vi "分层图显示1.1.vi"(11 "IN":string) -> (3 "OUT":string)   [LabVIEW 2016]
uses:
  <vilib>/Utility/file.llb/Read Delimited Spreadsheet (DBL).vi
panel:
  out "导入进度":u8(slide) scale=0.0..100.0
  in  "min":dbl format="%#_4e"
  in  "max":dbl format="%#_4e"
  in  "ESC":bool
  out "分层图":dbl[][](graph)
  in  "NEXT":bool
  in  "层数:":i32
  out "数组":dbl[][][](array[numeric])
  # "强度表"
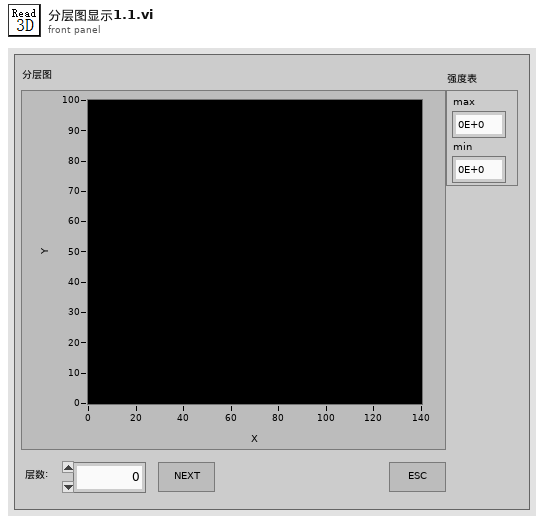
[diagram p1: front panel]
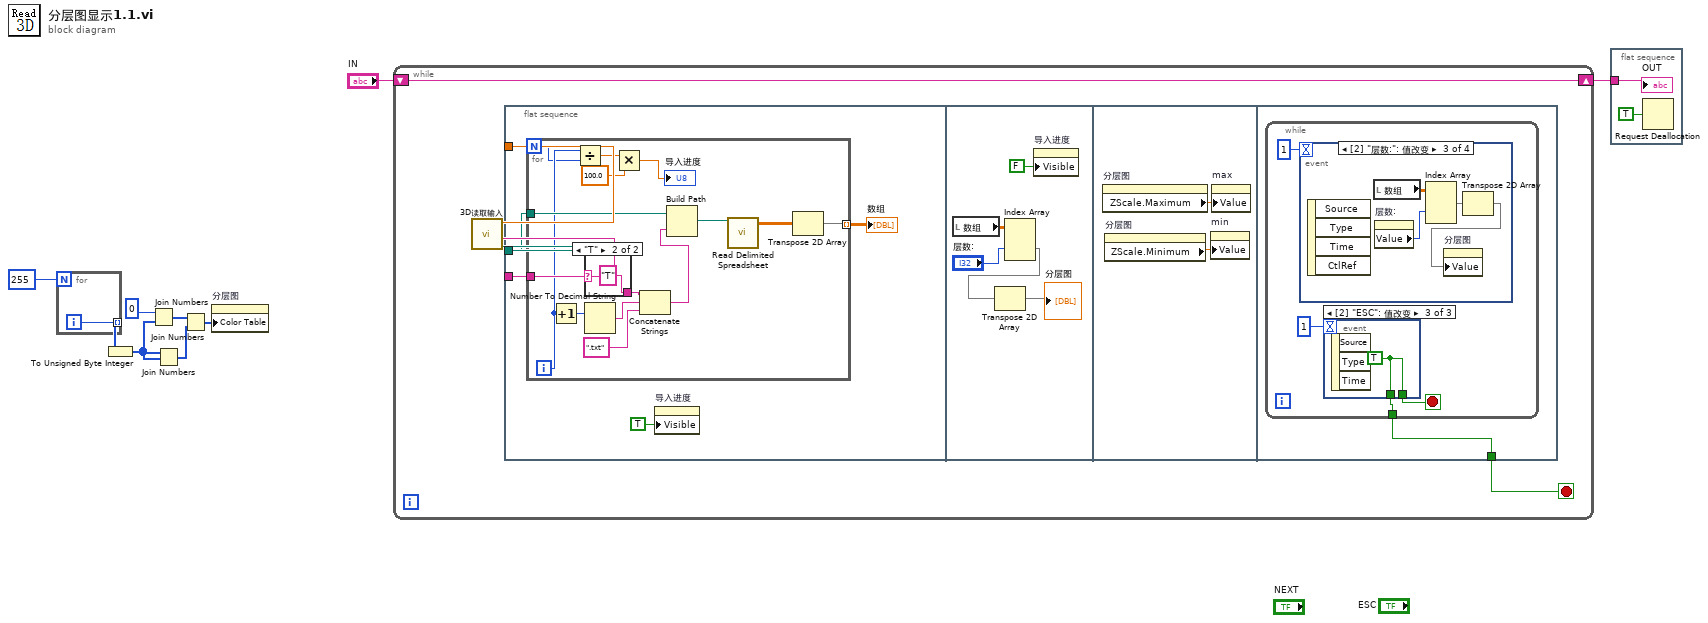
[diagram p0: block diagram]
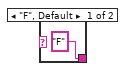
[diagram p2: hidden frame]
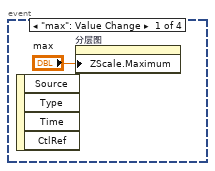
[diagram p3: hidden frame]
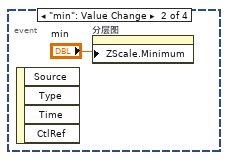
[diagram p4: hidden frame]
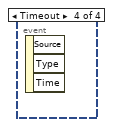
[diagram p5: hidden frame]
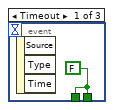
[diagram p6: hidden frame]
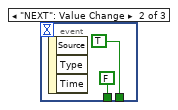
[diagram p7: hidden frame]
diagram:
  n1 = for {
    N: 255 -> [_]
    tunnel: [w10] -> w7 mode=indexing
    i -> [w10]
  }
  n2 = To Unsigned Byte Integer(number=w7) -> (unsigned 8bit integer=w4:u8[])
  n3 = Join Numbers(hi=u16 0, lo=w4) -> ((hi.lo)=w6:u32[])
  n4 = Join Numbers(hi=w4, lo=w4) -> ((hi.lo)=w3:u16[])
  n5 = Join Numbers(hi=w6, lo=w3) -> ((hi.lo)=w2:u64[])
  n6 = property on="分层图" class="IntGraph (严格)"("Color Table"=w2) -> ()  [unwired: 2 in, 2 out]
  n7 = while {
    shift-right: [w15] -> w8
    shift-left: "IN" -> [w15]
    stop <- w14 stop-if-true
    n8 = call "3D读取输入.vi"() -> ("文件读取路径"=w11:path, "时域谱or频域谱"=w12:string, "行总数"=w13:dbl)  [unwired: 9 in]
    n9 = flat-sequence {
      tunnel: w13 -> [w19]
      tunnel: w12 -> [w18]
      tunnel: w11 -> [w17]
      tunnel: [w45] -> w14
      frame #0 {
        n10 = for {
          N: w19 -> [w24]
          tunnel: [w34] -> w20 mode=indexing
          tunnel: w18 -> [w27]
          tunnel: w17 -> [w26]
          i -> [w25]
          n11 = Increment(x=w25) -> (x+1=w30:i32)
          n12 = Divide(x=w25, y=w24) -> (x/y=w23:dbl)
          n13 = case shown="\"T\"" w27 {
            tunnel: ["F" "T"] -> w32
            frame "F", Default {
            }
            frame "T" {
            }
          }
          n14 = Number To Decimal String(number=w30) -> (decimal integer string=w29:string)  [unwired: 1 in]
          n15 = Multiply(x=w23, y=100.0) -> (x*y=→"导入进度":dbl)
          n16 = Concatenate Strings(w32, w29, ".txt") -> (w31:string)
          n17 = Build Path(base path=w26, name or relative path=w31) -> (appended path=w33:path)
          n18 = call-poly <vilib>:"Read Delimited Spreadsheet.vi"("file path (dialog if empty)"=w33) -> ("all rows"=w35:dbl[][])  [unwired: 9 in, 5 out]
          n19 = Transpose 2D Array(2D array=w35) -> (transposed array=w34:dbl[][])
        }
        "数组" <- w20
        n20 = property on="导入进度" class="Slide (严格)"("Visible"=TRUE ("可见")) -> ()  [unwired: 2 in, 2 out]
      }
      frame #1 {
        n21 = local read "数组"() -> (w41:dbl[][][])
        n22 = Index Array(array=w41, index (dim 1)="层数:") -> (element=w39:dbl[][])  [unwired: 2 in]
        n23 = Transpose 2D Array(2D array=w39) -> (transposed array=→"分层图":dbl[][])
        n24 = property on="导入进度" class="Slide (严格)"("Visible"=FALSE ("可见")) -> ()  [unwired: 2 in, 2 out]
      }
      frame #2 {
        n25 = property on="分层图" class="IntGraph (严格)"() -> ("ZScale.Maximum"=w43:dbl)  [unwired: 2 in, 2 out]
        n26 = property on="分层图" class="IntGraph (严格)"() -> ("ZScale.Minimum"=w44:dbl)  [unwired: 2 in, 2 out]
        n27 = property on="min" class="DigNum (严格)"("Value"=w44) -> ()  [unwired: 2 in, 2 out]
        n28 = property on="max" class="DigNum (严格)"("Value"=w43) -> ()  [unwired: 2 in, 2 out]
      }
      frame #3 {
        n29 = while {
          tunnel: [w48] -> w45
          stop <- w49 stop-if-true
          n30 = event shown="[2] \"层数:\": 值改变" {
            selector: _ -> [_ _ _ _]
            dyn-events: _ -> [_ _ _ _]
            timeout: 1 -> [_ _ _ _]
            event "max": Value Change {
              n31 = event-data() -> ()  [unwired: 1 in, 4 out]
              n32 = property on="分层图" class="IntGraph (严格)"("ZScale.Maximum"="max") -> ()  [unwired: 2 in, 2 out]
            }
            event "min": Value Change {
              n33 = event-data() -> ()  [unwired: 1 in, 4 out]
              n34 = property on="分层图" class="IntGraph (严格)"("ZScale.Minimum"="min") -> ()  [unwired: 2 in, 2 out]
            }
            event "层数:": Value Change {
              n35 = event-data() -> ()  [unwired: 1 in, 4 out]
              n36 = local read "数组"() -> (w54:dbl[][][])
              n37 = property on="层数:" class="DigNum (严格)"() -> ("Value"=w55:i32)  [unwired: 2 in, 2 out]
              n38 = Index Array(array=w54, index (dim 1)=w55) -> (element=w53:dbl[][])  [unwired: 2 in]
              n39 = Transpose 2D Array(2D array=w53) -> (transposed array=w52:dbl[][])
              n40 = property on="分层图" class="IntGraph (严格)"("Value"=w52) -> ()  [unwired: 2 in, 2 out]
            }
            event Timeout {
              n41 = event-data() -> ()  [unwired: 1 in, 3 out]
            }
          }
          n42 = event shown="[2] \"ESC\": 值改变" {
            selector: _ -> [_ _ _]
            dyn-events: _ -> [_ _ _]
            timeout: 1 -> [_ _ _]
            tunnel: [w56 TRUE w59] -> w49
            tunnel: [w56 FALSE w59] -> w48
            event Timeout {
              w56 = FALSE
              n43 = event-data() -> ()  [unwired: 1 in, 3 out]
            }
            event "NEXT": Value Change {
              n44 = event-data() -> ()  [unwired: 1 in, 3 out]
            }
            event "ESC": Value Change {
              w59 = TRUE
              n45 = event-data() -> ()  [unwired: 1 in, 3 out]
            }
          }
        }
      }
    }
  }
  n46 = flat-sequence {
    tunnel: w8 -> [w61]
    frame #0 {
      n47 = Request Deallocation(TRUE ("标志")) -> ()
      "OUT" <- w61
    }
  }
